vi "weight_experimental5.vi"(9 "Stop read":bool, 10 "N_points":i32=180, 11 "PV weight":dbl caption="g" format="%#.0f") -> (0 "Weight 3":dbl format="%#.0f", 2 "Weight 2":dbl format="%#.0f", 5 "Weight 1":dbl format="%#.0f")   [LabVIEW 2019]
uses:
  <vilib>/Analysis/baseanly.llb/Mean (DBL).vi
  Logik/fronts.vi
  Trigers/RS.vi
  Reg/PID Timing Estimation.vi
  <vilib>/Analysis/NI_AALBase.lvlib
  Timer Delay/Timers.lvlib
  <vilib>/Analysis/3filter.llb/Filter Passband Type.ctl
  Reg/control.lvlib
  <vilib>/Analysis/3filter.llb/Butterworth Filter (DBL).vi
panel:
  in  "Tab Control":T1(tab)
  in  "Tare":dbl caption="g" format="%#.0f"
  in  "k":dbl=1.0 caption="g" format="%#.3f"
  # "Усреднение за 1 мин"
  # "(расход)"
  # "Усреднение за 3 мин"
  # "(расход)"
  # "Вес тары\n(полностью очистить бункер от продукта\nи запомнить PV weight или ввести вручную)."
  # "Вес тары\n(ввести фактический вес без учета тары\nили ввести k вручную)"
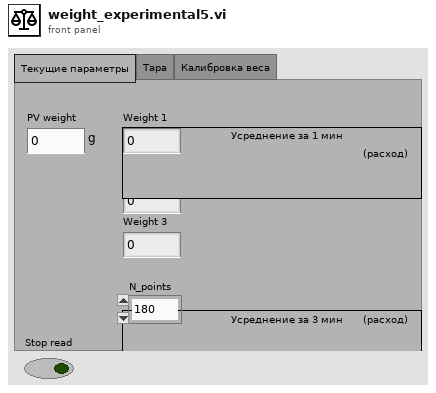
[diagram p1: front panel]
types:
  T1 = enum32{"Текущие параметры", "Тара", "Калибровка веса"}
  T2 = typedef "NI_AALBase.lvlib/Filter Passband Type.ctl" = enum32{"Lowpass", "Highpass", "Bandpass", "Bandstop"}
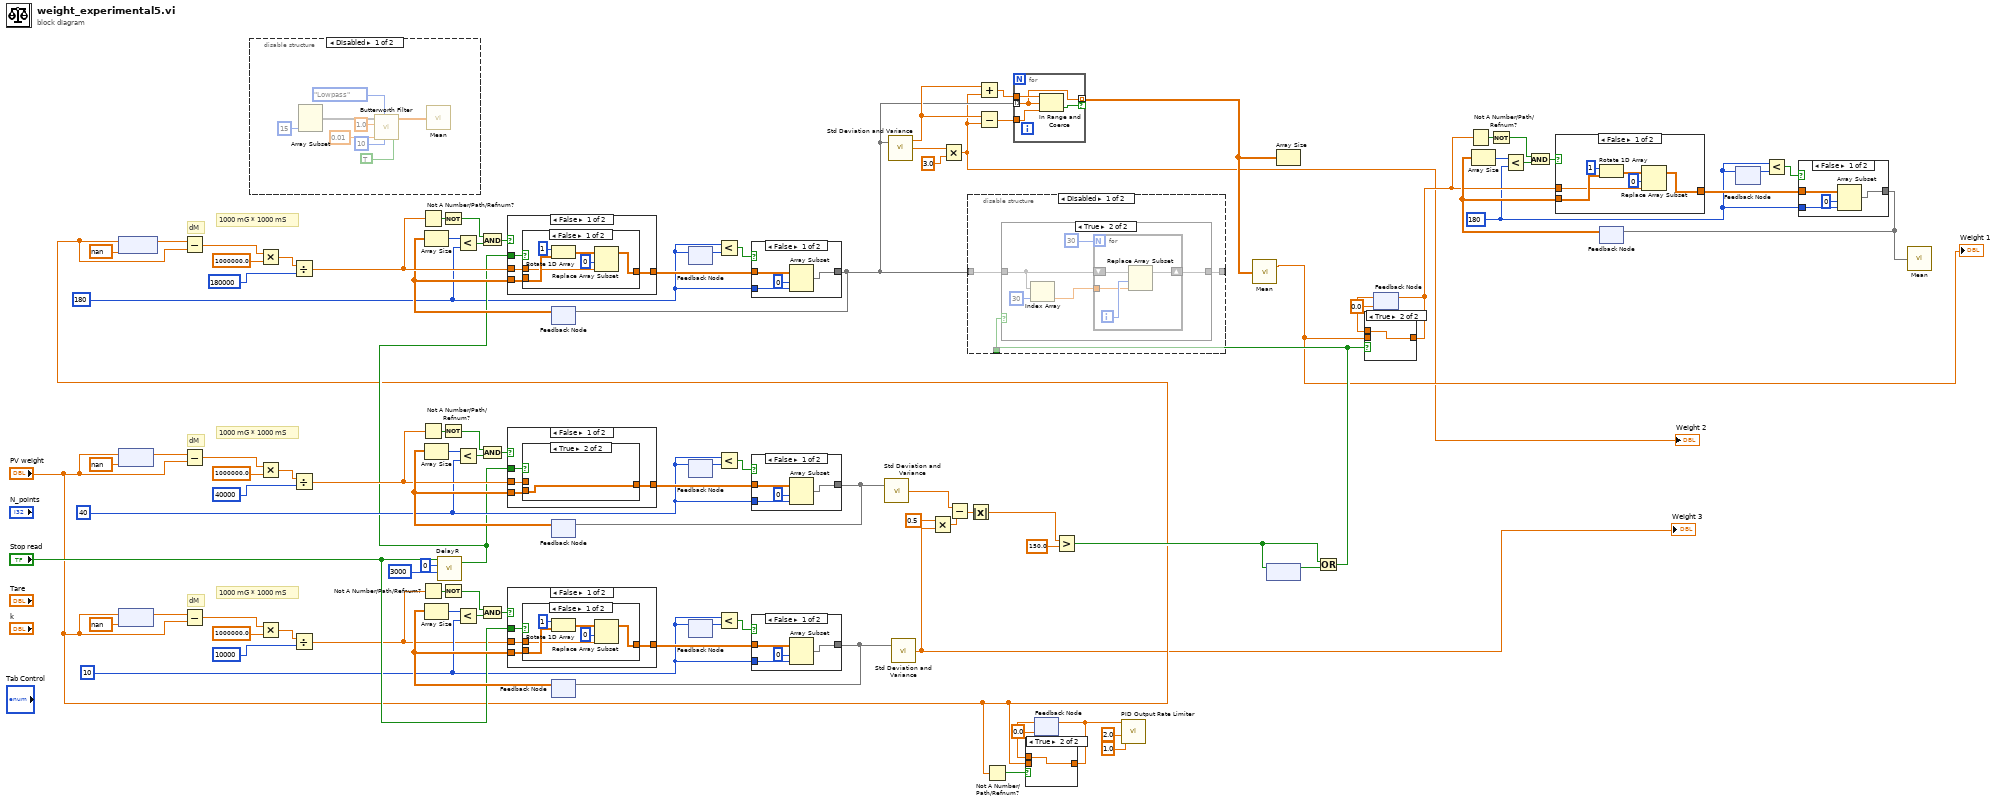
[diagram p0: block diagram]
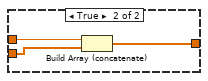
[diagram p3: hidden frame]
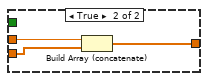
[diagram p9: hidden frame]
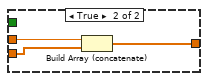
[diagram p13: hidden frame]
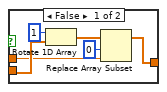
[diagram p16: hidden frame]
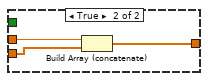
[diagram p17: hidden frame]
diagram:
  w13 = 180 ("N_points")
  w14 = 180 ("N_points")
  w52 = 40 ("N_points")
  w62 = 10 ("N_points")
  # "1000 mG * 1000 mS"
  # "dM"
  # "1000 mG * 1000 mS"
  # "dM"
  # "1000 mG * 1000 mS"
  # "dM"
  n1 = feedback #1(nan) -> (w47:dbl)
  n2 = feedback-in #1("PV weight") -> ()
  n3 = feedback #2(nan) -> (w84:dbl)
  n4 = feedback-in #2("PV weight") -> ()
  n5 = feedback #3(nan) -> (w75:dbl)
  n6 = feedback-in #3("PV weight") -> ()
  n7 = Subtract(x=w47, y="PV weight") -> (x-y=w50:dbl)
  n8 = Subtract(x=w84, y="PV weight") -> (x-y=w81:dbl)
  n9 = Subtract(x=w75, y="PV weight") -> (x-y=w78:dbl)
  n10 = disable-structure shown="Disabled" {
    frame Disabled {
      n11 = Array Subset(length=15) -> (w99:void[])  [unwired: 2 in]
      n12 = call-poly <vilib>:"Butterworth Filter.vi"("init/cont (init:F)"=TRUE, "order"=10, "filter type"=Filter_Passband_Type."Lowpass", "low cutoff freq: fl"=0.01, "sampling freq: fs"=1.0, "X"=w99) -> ("Filtered X"=w98:dbl[])  [unwired: 2 in, 1 out]
      n13 = call-poly <vilib>:"Mean.vi"("X"=w98) -> ()  [unwired: 2 out]
    }
    frame Enabled {
    }
  }
  n14 = Multiply(x=w50, y=1000000.0) -> (x*y=w48:dbl)
  n15 = Multiply(x=w81, y=1000000.0) -> (x*y=w83:dbl)
  n16 = Multiply(x=w78, y=1000000.0) -> (x*y=w76:dbl)
  n17 = Divide(x=w48, y=u32 180000 ("millisecond timer value")) -> (x/y=w51:dbl)
  n18 = Divide(x=w83, y=u32 40000 ("millisecond timer value")) -> (x/y=w80:dbl)
  n19 = Divide(x=w76, y=u32 10000 ("millisecond timer value")) -> (x/y=w56:dbl)
  n20 = Not A Number/Path/Refnum?(number/path/refnum=w51) -> (NaN/Path/Refnum?=w40:bool)
  n21 = Not A Number/Path/Refnum?(number/path/refnum=w80) -> (NaN/Path/Refnum?=w93:bool)
  n22 = Not A Number/Path/Refnum?(number/path/refnum=w56) -> (NaN/Path/Refnum?=w68:bool)
  n23 = call "DelayR.vi"("DelayOff"=u32 3000, "DelayOn"=u32 0, "In"="Stop read") -> ("Out"=w35:bool)  [unwired: 1 in, 1 out]
  n24 = Not(x=w40) -> (.not. x?=w41:bool)
  n25 = Not(x=w93) -> (.not. x?=w92:bool)
  n26 = Not(x=w68) -> (.not. x?=w69:bool)
  n27 = feedback #4() -> (w37:dbl[])  [unwired: 1 in]
  n28 = Array Size(array=w37) -> (size(s)=w36:i32)
  n29 = Less?(x=w36, y=w14) -> (x < y?=w38:bool)
  n30 = And(x=w41, y=w38) -> (x .and. y?=w39:bool)
  n31 = case shown="False" w39 {
    tunnel: [w107 w118] -> w42
    tunnel: w51 -> [w108 w119]
    tunnel: w37 -> [w109 w117]
    tunnel: w35 -> [w106 _]
    frame False {
      n32 = case shown="False" w106 {
        tunnel: w109 -> [w112 w116]
        tunnel: w108 -> [w111 _]
        tunnel: [w110 w116] -> w107
        frame False {
          n33 = Rotate 1D Array(1:w112, 2:1 ("n")) -> (0:w114:dbl[])
          n34 = Replace Array Subset(array=w114, new element=w111, index=0) -> (w110:dbl[])
        }
        frame True {
        }
      }
    }
    frame True {
      n35 = Build Array (concatenate)(w119, w117) -> (w118:dbl[])
    }
  }
  n36 = feedback #5() -> (w96:dbl[])  [unwired: 1 in]
  n37 = Array Size(array=w96) -> (size(s)=w97:i32)
  n38 = Less?(x=w97, y=w52) -> (x < y?=w95:bool)
  n39 = And(x=w92, y=w95) -> (x .and. y?=w94:bool)
  n40 = case shown="False" w94 {
    tunnel: [w121 w132] -> w91
    tunnel: w80 -> [w122 w133]
    tunnel: w96 -> [w123 w131]
    tunnel: w35 -> [w120 _]
    frame False {
      n41 = case shown="True" w120 {
        tunnel: w123 -> [w126 w130]
        tunnel: w122 -> [w125 _]
        tunnel: [w124 w130] -> w121
        frame False {
          n42 = Rotate 1D Array(1:w126, 2:1 ("n")) -> (0:w128:dbl[])
          n43 = Replace Array Subset(array=w128, new element=w125, index=0) -> (w124:dbl[])
        }
        frame True {
        }
      }
    }
    frame True {
      n44 = Build Array (concatenate)(w133, w131) -> (w132:dbl[])
    }
  }
  n45 = feedback #6() -> (w65:dbl[])  [unwired: 1 in]
  n46 = Array Size(array=w65) -> (size(s)=w64:i32)
  n47 = Less?(x=w64, y=w62) -> (x < y?=w66:bool)
  n48 = And(x=w69, y=w66) -> (x .and. y?=w67:bool)
  n49 = case shown="False" w67 {
    tunnel: [w135 w146] -> w70
    tunnel: w56 -> [w136 w147]
    tunnel: w65 -> [w137 w145]
    tunnel: "Stop read" -> [w134 _]
    frame False {
      n50 = case shown="False" w134 {
        tunnel: w137 -> [w140 w144]
        tunnel: w136 -> [w139 _]
        tunnel: [w138 w144] -> w135
        frame False {
          n51 = Rotate 1D Array(1:w140, 2:1 ("n")) -> (0:w142:dbl[])
          n52 = Replace Array Subset(array=w142, new element=w139, index=0) -> (w138:dbl[])
        }
        frame True {
        }
      }
    }
    frame True {
      n53 = Build Array (concatenate)(w147, w145) -> (w146:dbl[])
    }
  }
  n54 = feedback #7() -> (w43:i32)  [unwired: 1 in]
  n55 = feedback-in #7(w14) -> ()
  n56 = feedback #8() -> (w90:i32)  [unwired: 1 in]
  n57 = feedback-in #8(w52) -> ()
  n58 = feedback #9() -> (w71:i32)  [unwired: 1 in]
  n59 = feedback-in #9(w62) -> ()
  n60 = Less?(x=w14, y=w43) -> (x < y?=w44:bool)
  n61 = Less?(x=w52, y=w90) -> (x < y?=w89:bool)
  n62 = Less?(x=w62, y=w71) -> (x < y?=w72:bool)
  n63 = case shown="False" w44 {
    tunnel: [w150 w152] -> w5
    tunnel: w42 -> [w151 w152]
    tunnel: w14 -> [w148 _]
    frame False {
      n64 = Array Subset(array=w151, index=0, length=w148) -> (w150:dbl[])
    }
    frame True {
    }
  }
  n65 = feedback-in #4(w5) -> ()
  n66 = case shown="False" w89 {
    tunnel: [w155 w157] -> w79
    tunnel: w91 -> [w156 w157]
    tunnel: w52 -> [w153 _]
    frame False {
      n67 = Array Subset(array=w156, index=0, length=w153) -> (w155:dbl[])
    }
    frame True {
    }
  }
  n68 = feedback-in #5(w79) -> ()
  n69 = case shown="False" w72 {
    tunnel: [w160 w162] -> w61
    tunnel: w70 -> [w161 w162]
    tunnel: w62 -> [w158 _]
    frame False {
      n70 = Array Subset(array=w161, index=0, length=w158) -> (w160:dbl[])
    }
    frame True {
    }
  }
  n71 = feedback-in #6(w61) -> ()
  n72 = call <vilib>:"Std Deviation and Variance.vi"("X"=w79) -> ("standard deviation"=w32:dbl)  [unwired: 1 in, 2 out]
  n73 = call <vilib>:"Std Deviation and Variance.vi"("X"=w5) -> ("mean"=w10:dbl, "standard deviation"=w7:dbl)  [unwired: 1 in, 1 out]
  n74 = call <vilib>:"Std Deviation and Variance.vi"("X"=w61) -> ("standard deviation"=w1:dbl)  [unwired: 1 in, 2 out]
  "Weight 3" <- w1
  n75 = Multiply(x=0.5, y=w1) -> (x*y=w31:dbl)
  n76 = Multiply(x=w7, y=3.0) -> (x*y=w2:dbl)
  "Weight 2" <- w2
  n77 = Subtract(x=w32, y=w31) -> (x-y=w29:dbl)
  n78 = Absolute Value(x=w29) -> (abs(x)=w28:dbl)
  n79 = Add(x=w10, y=w2) -> (x+y=w9:dbl)
  n80 = Subtract(x=w10, y=w2) -> (x-y=w8:dbl)
  n81 = Not A Number/Path/Refnum?(number/path/refnum="PV weight") -> (NaN/Path/Refnum?=w57:bool)
  n82 = for {
    tunnel: w5 -> [w163] mode=indexing
    tunnel: w9 -> [w166]
    tunnel: w8 -> [w165]
    tunnel: [w163] -> w3 mode=indexing if=w164
    n83 = In Range and Coerce(upper limit=w166, x=w163, lower limit=w165) -> (In Range?=w164:bool)  [unwired: 1 out]
  }
  n84 = feedback #10(0.0) -> (w58:dbl)
  n85 = case shown="True" w57 {
    tunnel: "PV weight" -> [w167 _]
    tunnel: [w167 w168] -> w54
    tunnel: w58 -> [_ w168]
    frame False {
    }
    frame True {
    }
  }
  n86 = feedback-in #10(w54) -> ()
  n87 = Greater?(x=w28, y=150.0) -> (0:w27:bool)
  n88 = call "PID Output Rate Limiter.vi"("dt (s)"=1.0, "output rate (EGU/s)"=2.0, "input (controller output)"=w54) -> ()  [unwired: 7 in, 2 out]
  n89 = call-poly <vilib>:"Mean.vi"("X"=w3) -> ("mean"=w11:dbl)  [unwired: 1 out]
  "Weight 1" <- w11
  n90 = feedback #11() -> (w26:bool)  [unwired: 1 in]
  n91 = feedback-in #11(w27) -> ()
  n92 = Array Size(array=w3) -> ()  [unwired: 1 out]
  n93 = Or(x=w27, y=w26) -> (x .or. y?=w25:bool)
  n94 = disable-structure shown="Disabled" {
    disable-tunnel: w5 -> [w171 w182]
    disable-tunnel: [w170 w182] -> _
    disable-tunnel: w25 -> [w169 _]
    frame Disabled {
      n95 = case shown="True" w169 {
        tunnel: w171 -> [w172 w177]
        tunnel: [w172 w173] -> w170
        frame False {
        }
        frame True {
          n96 = Index Array(array=w177, index=30) -> (element=w174:dbl)
          n97 = for {
            N: 30 ("x") -> [_]
            shift-right: [w179] -> w173
            shift-left: w177 -> [w181]
            tunnel: w174 -> [w178]
            i -> [w180]
            n98 = Replace Array Subset(array=w181, new element=w178, index=w180) -> (w179:dbl[])
          }
        }
      }
    }
    frame Enabled {
    }
  }
  n99 = feedback #12(0.0) -> (w34:dbl)
  n100 = case shown="True" w25 {
    tunnel: w11 -> [w183 _]
    tunnel: [w183 w184] -> w15
    tunnel: w34 -> [_ w184]
    frame False {
    }
    frame True {
    }
  }
  n101 = feedback-in #12(w15) -> ()
  n102 = Not A Number/Path/Refnum?(number/path/refnum=w15) -> (NaN/Path/Refnum?=w20:bool)
  n103 = Not(x=w20) -> (.not. x?=w21:bool)
  n104 = feedback #13() -> (w17:dbl[])  [unwired: 1 in]
  n105 = Array Size(array=w17) -> (size(s)=w16:i32)
  n106 = Less?(x=w16, y=w13) -> (x < y?=w18:bool)
  n107 = And(x=w21, y=w18) -> (x .and. y?=w19:bool)
  n108 = case shown="False" w19 {
    tunnel: [w188 w192] -> w22
    tunnel: w15 -> [w189 w193]
    tunnel: w17 -> [w190 w191]
    frame False {
      n109 = Rotate 1D Array(1:w190, 2:1 ("n")) -> (0:w186:dbl[])
      n110 = Replace Array Subset(array=w186, new element=w189, index=0) -> (w188:dbl[])
    }
    frame True {
      n111 = Build Array (concatenate)(w193, w191) -> (w192:dbl[])
    }
  }
  n112 = feedback #14() -> (w23:i32)  [unwired: 1 in]
  n113 = feedback-in #14(w13) -> ()
  n114 = Less?(x=w13, y=w23) -> (x < y?=w24:bool)
  n115 = case shown="False" w24 {
    tunnel: [w196 w198] -> w12
    tunnel: w22 -> [w197 w198]
    tunnel: w13 -> [w194 _]
    frame False {
      n116 = Array Subset(array=w197, index=0, length=w194) -> (w196:dbl[])
    }
    frame True {
    }
  }
  n117 = feedback-in #13(w12) -> ()
  n118 = call-poly <vilib>:"Mean.vi"("X"=w12) -> ()  [unwired: 2 out]
